vi "R&W_Moudle.vi"() -> ()   [LabVIEW 2019]
uses:
  <vilib>/myRIO/Instrument Drivers/Onboard IO/UART/typedef/VISA Configuration.ctl
  <vilib>/Instr/_visa.llb/VISA Configure Serial Port (Instr).vi
  <vilib>/myRIO/Instrument Drivers/Onboard IO/UART/UART.lvlib
panel:
  out "Characters to Read":string
  in  "read":bool
  in  "Write":bool
  out "error out":errorcluster
  in  "error in (no error)":errorcluster
  in  "Characters to Write":string
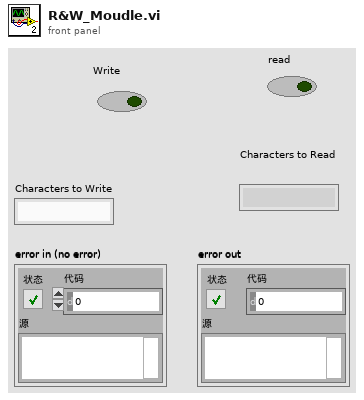
[diagram p1: front panel]
types:
  T1 = typedef "UART.lvlib/VISA Configuration.ctl" = cluster{"baud rate (9600)":u32, "data bits (8)":u16, "parity (0:none)":enum16{"None", "Odd", "Even", "Mark", "Space"}, "stop bits (10: 1 bit)":u16, "flow control (0:none)":u16, "termination char\n(0xA = '\\n' = LF) ":u8, "Enable Termination\nChar (T)":bool, "timeout (10sec)":u32}
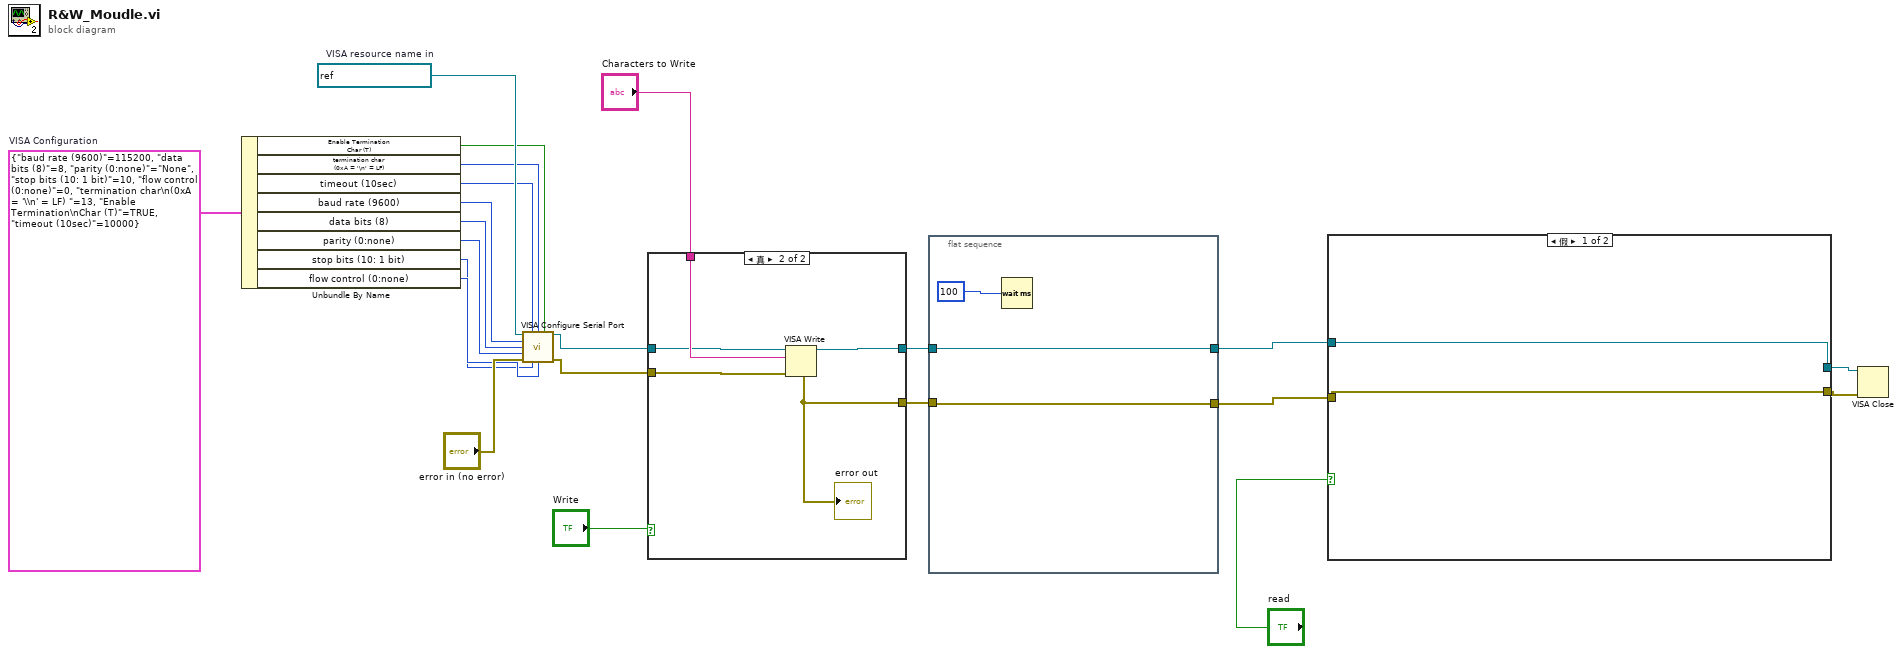
[diagram p0: block diagram]
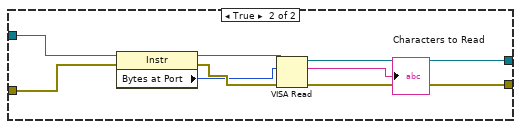
[diagram p2: hidden frame]
diagram:
  w21 = T1 {"baud rate (9600)"=115200, "data bits (8)"=8, "parity (0:none)"=enum."None", "stop bits (10: 1 bit)"=10, "flow control (0:none)"=0, "termination char\n(0xA = '\\n' = LF) "=13, "Enable Termination\nChar (T)"=TRUE, "timeout (10sec)"=10000}  # VISA Configuration
  w22 = refnum<visa-resource-name> "ASRL1::INSTR"  # VISA resource name in
  n1 = Unbundle By Name(w21) -> ("Enable Termination\nChar (T)"=w19:bool, "termination char\n(0xA = '\\n' = LF)"=w18:u8, "timeout (10sec)"=w17:u32, "baud rate (9600)"=w12:u32, "data bits (8)"=w13:u16, "parity (0:none)"=w14:enum16{"None", "Odd", "Even", "Mark", "Space"}, "stop bits (10: 1 bit)"=w15:u16, "flow control (0:none)"=w16:u16)
  n2 = call-poly "VISA Configure Serial Port"("VISA resource name"=w22, "timeout (10sec)"=w17, "termination char\n(0xA = '\\n' = LF)"=w18, "Enable Termination\nChar (T)"=w19, "baud rate (9600)"=w12, "data bits (8)"=w13, "parity (0:none)"=w14, "error in (no error)"="error in (no error)", "stop bits (10: 1 bit)"=w15, "flow control (0:none)"=w16) -> ("VISA resource name out"=w9:refnum<visa-resource-name>, "error out"=w11:errorcluster)  [unwired: 4 in]
  n3 = case shown="真" "Write" {
    tunnel: w11 -> [w23 w29]
    tunnel: "Characters to Write" -> [_ w28]
    tunnel: w9 -> [w24 w27]
    tunnel: [w24 w26] -> w7
    tunnel: [w23 w25] -> w5
    frame False {
    }
    frame True {
      n4 = VISA Write(VISA resource name=w27, write buffer=w28, error in (no error)=w29) -> (VISA resource name out=w26:refnum<visa-resource-name>, error out=w25:errorcluster)  [unwired: 1 out]
      "error out" <- w25
    }
  }
  n5 = flat-sequence {
    tunnel: w7 -> [w31]
    tunnel: [w31] -> w6
    tunnel: [w30] -> w4
    tunnel: w5 -> [w30]
    frame #0 {
      n6 = Wait (ms)(milliseconds to wait=u32 100 ("等待时间（毫秒）")) -> ()  [unwired: 1 out]
    }
  }
  n7 = case shown="假" "read" {
    tunnel: w6 -> [w34 w42]
    tunnel: w4 -> [w33 w41]
    tunnel: [w34 w36] -> w2
    tunnel: [w33 w35] -> w1
    frame False {
    }
    frame True {
      n8 = property class="Instr"(reference=w42, error in=w41) -> (reference out=w40:refnum<visa-resource-name>, error out=w39:errorcluster, "Bytes at Port"=w38:u32)
      n9 = VISA Read(VISA resource name=w40, byte count=w38, error in (no error)=w39) -> (VISA resource name out=w36:refnum<visa-resource-name>, read buffer=→"Characters to Read":string, error out=w35:errorcluster)  [unwired: 1 out]
    }
  }
  n10 = VISA Close(VISA resource name=w2, error in (no error)=w1) -> ()  [unwired: 1 out]
